vi "6221-6229_sample_rate.vi"(1 "# of output channels":i32) -> (0 "Sampling rate":dbl)   [LabVIEW 2013]
uses:
  Instance           1 29Saved   6221-6229_sample_rate .vi
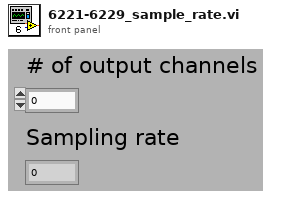
[diagram p1: front panel]
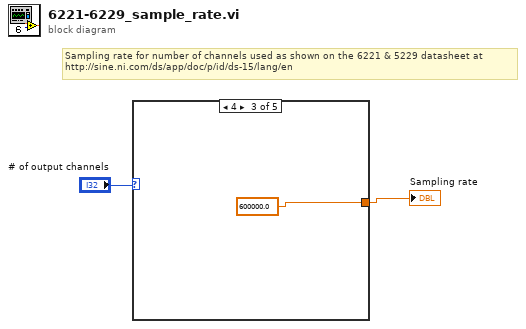
[diagram p0: block diagram]
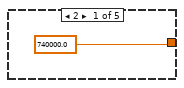
[diagram p2: hidden frame]
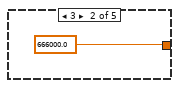
[diagram p3: hidden frame]
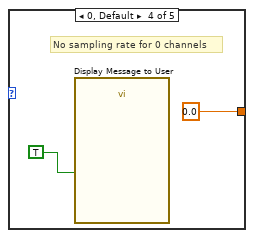
[diagram p4: hidden frame]
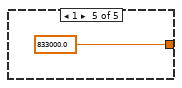
[diagram p5: hidden frame]
diagram:
  # "Sampling rate for number of channels used as shown on the 6221 & 5229 datasheet at\nhttp://sine.ni.com/ds/app/doc/p/id/ds-15/lang/en"
  n1 = case shown="4" "# of output channels" {
    tunnel: [740000.0 666000.0 600000.0 0.0 833000.0] -> w1
    frame 2 {
    }
    frame 3 {
    }
    frame 4 {
    }
    frame 0, Default {
      # "No sampling rate for 0 channels"
      n2 = call "Display Message to User"("Enable"=TRUE) -> ()  [unwired: 9 in, 2 out]
    }
    frame 1 {
    }
  }
  "Sampling rate" <- w1
